vi "Mappa Aplus into WT cluster.vi"(11 "Cluster in":T2) -> (3 "MISURE WT":T1)   [LabVIEW 2019]
uses:
  TypeDef/MISURE WT.ctl
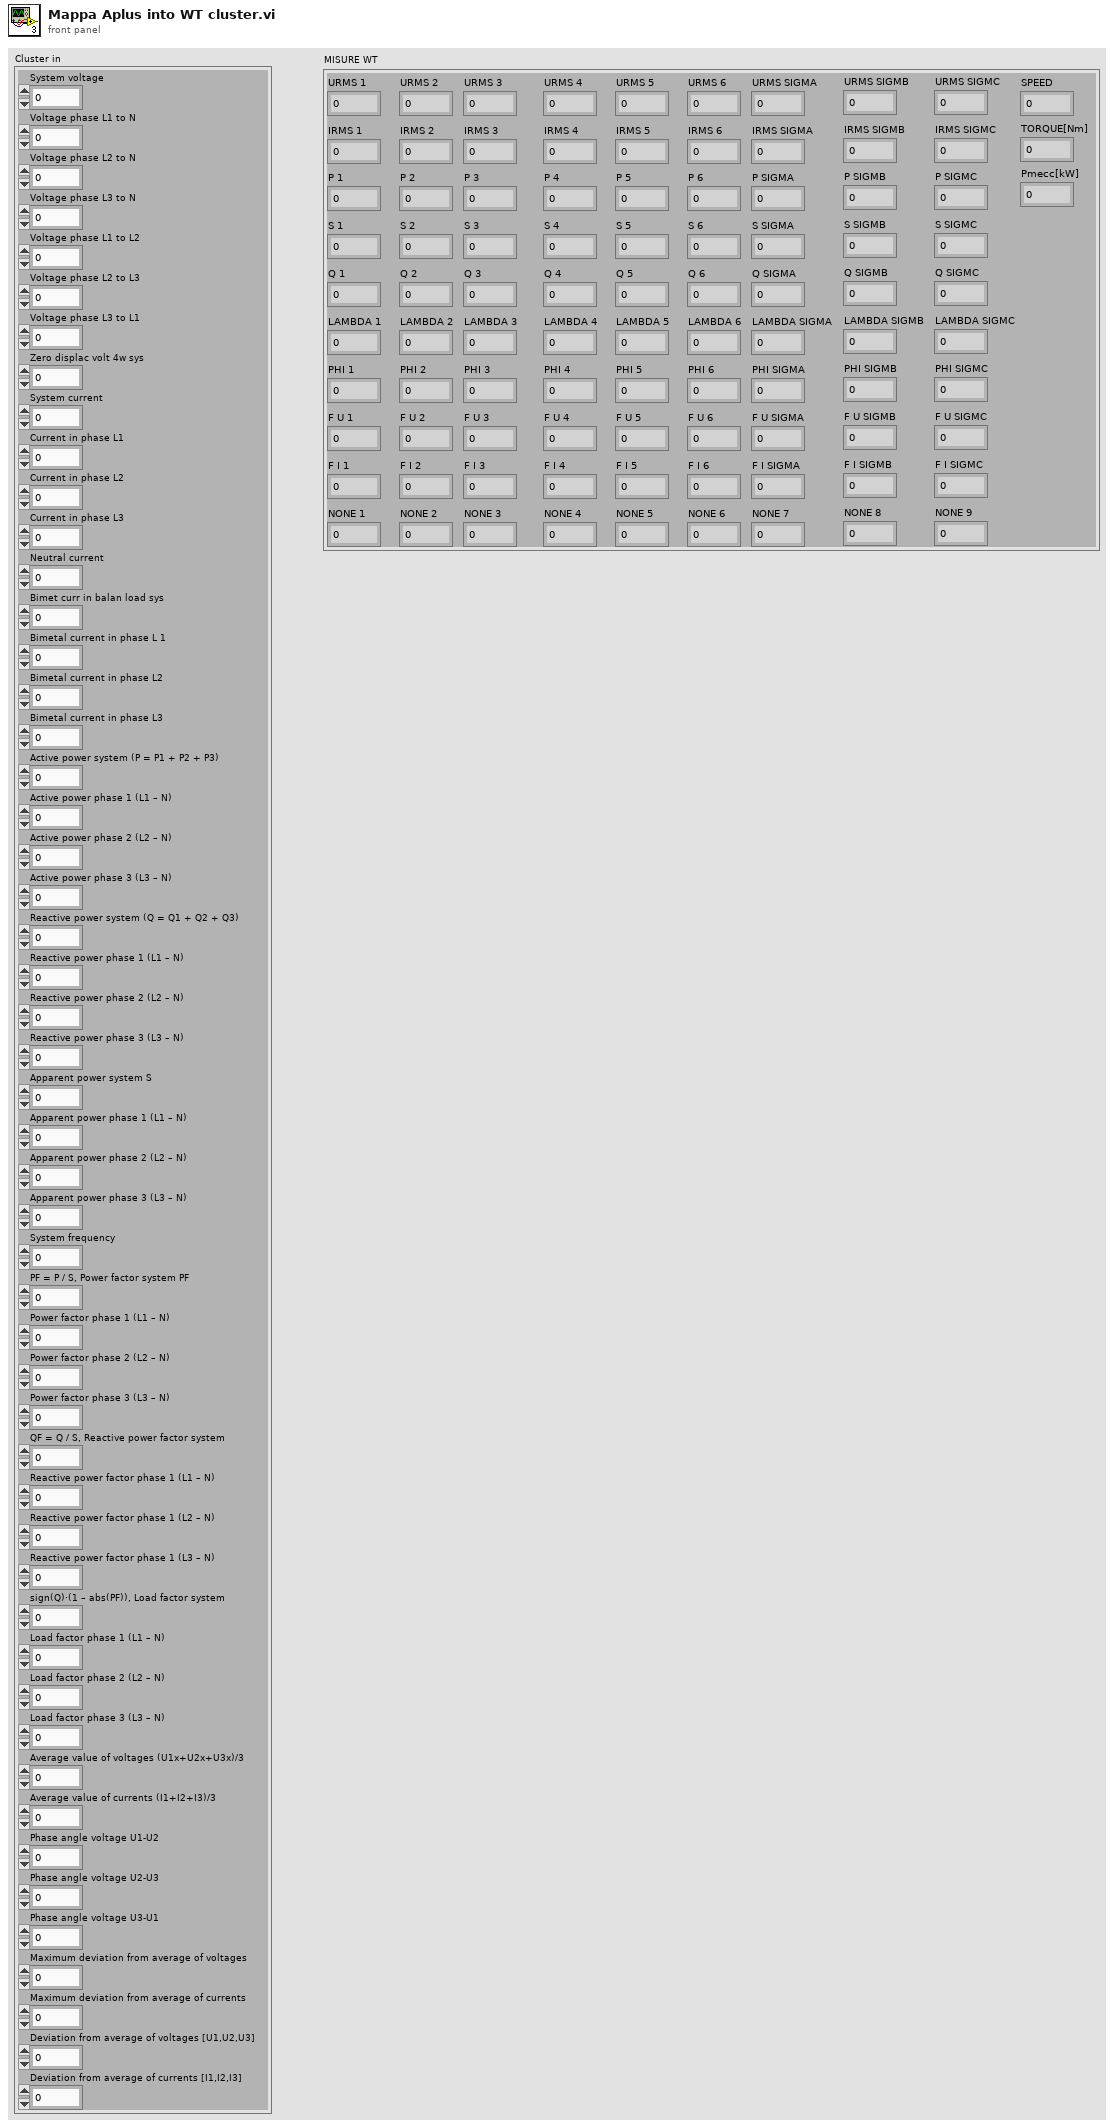
[diagram p1: front panel]
types:
  T1 = typedef "MISURE WT.ctl" = cluster{"URMS 1":dbl, "IRMS 1":dbl, "P 1":dbl, "S 1":dbl, "Q 1":dbl, "LAMBDA 1":dbl, "PHI 1":dbl, "F U 1":dbl, "F I 1":dbl, "NONE 1":dbl, "URMS 2":dbl, "IRMS 2":dbl, "P 2":dbl, "S 2":dbl, "Q 2":dbl, "LAMBDA 2":dbl, "PHI 2":dbl, "F U 2":dbl, "F I 2":dbl, "NONE 2":dbl, "URMS 3":dbl, "IRMS 3":dbl, "P 3":dbl, "S 3":dbl, "Q 3":dbl, "LAMBDA 3":dbl, "PHI 3":dbl, "F U 3":dbl, "F I 3":dbl, "NONE 3":dbl, "URMS 4":dbl, "IRMS 4":dbl, "P 4":dbl, "S 4":dbl, "Q 4":dbl, "LAMBDA 4":dbl, "PHI 4":dbl, "F U 4":dbl, "F I 4":dbl, "NONE 4":dbl, "URMS 5":dbl, "IRMS 5":dbl, "P 5":dbl, "S 5":dbl, "Q 5":dbl, "LAMBDA 5":dbl, "PHI 5":dbl, "F U 5":dbl, "F I 5":dbl, "NONE 5":dbl, "URMS 6":dbl, "IRMS 6":dbl, "P 6":dbl, "S 6":dbl, "Q 6":dbl, "LAMBDA 6":dbl, "PHI 6":dbl, "F U 6":dbl, "F I 6":dbl, "NONE 6":dbl, "URMS SIGMA":dbl, "IRMS SIGMA":dbl, "P SIGMA":dbl, "S SIGMA":dbl, "Q SIGMA":dbl, "LAMBDA SIGMA":dbl, "PHI SIGMA":dbl, "F U SIGMA":dbl, "F I SIGMA":dbl, "NONE 7":dbl, "URMS SIGMB":dbl, "IRMS SIGMB":dbl, "P SIGMB":dbl, "S SIGMB":dbl, "Q SIGMB":dbl, "LAMBDA SIGMB":dbl, "PHI SIGMB":dbl, "F U SIGMB":dbl, "F I SIGMB":dbl, "NONE 8":dbl, "URMS SIGMC":dbl, "IRMS SIGMC":dbl, "P SIGMC":dbl, "S SIGMC":dbl, "Q SIGMC":dbl, "LAMBDA SIGMC":dbl, "PHI SIGMC":dbl, "F U SIGMC":dbl, "F I SIGMC":dbl, "NONE 9":dbl, "SPEED":dbl, "TORQUE[Nm]":dbl, "Pmecc[kW]":dbl}
  T2 = cluster{"System voltage":dbl, "Voltage phase L1 to N":dbl, "Voltage phase L2 to N":dbl, "Voltage phase L3 to N":dbl, "Voltage phase L1 to L2":dbl, "Voltage phase L2 to L3":dbl, "Voltage phase L3 to L1":dbl, "Zero displac volt 4w sys":dbl, "System current":dbl, "Current in phase L1":dbl, "Current in phase L2":dbl, "Current in phase L3":dbl, "Neutral current":dbl, "Bimet curr in balan load sys":dbl, "Bimetal current in phase L 1":dbl, "Bimetal current in phase L2":dbl, "Bimetal current in phase L3":dbl, "Active power system (P = P1 + P2 + P3)":dbl, "Active power phase 1 (L1 – N)":dbl, "Active power phase 2 (L2 – N)":dbl, "Active power phase 3 (L3 – N)":dbl, "Reactive power system (Q = Q1 + Q2 + Q3)":dbl, "Reactive power phase 1 (L1 – N)":dbl, "Reactive power phase 2 (L2 – N)":dbl, "Reactive power phase 3 (L3 – N)":dbl, "Apparent power system S":dbl, "Apparent power phase 1 (L1 – N)":dbl, "Apparent power phase 2 (L2 – N)":dbl, "Apparent power phase 3 (L3 – N)":dbl, "System frequency":dbl, "PF = P / S, Power factor system PF":dbl, "Power factor phase 1 (L1 – N)":dbl, "Power factor phase 2 (L2 – N)":dbl, "Power factor phase 3 (L3 – N)":dbl, "QF = Q / S, Reactive power factor system":dbl, "Reactive power factor phase 1 (L1 – N)":dbl, "Reactive power factor phase 1 (L2 – N)":dbl, "Reactive power factor phase 1 (L3 – N)":dbl, "sign(Q)·(1 – abs(PF)), Load factor system":dbl, "Load factor phase 1 (L1 – N)":dbl, "Load factor phase 2 (L2 – N)":dbl, "Load factor phase 3 (L3 – N)":dbl, "Average value of voltages (U1x+U2x+U3x)/3":dbl, "Average value of currents (I1+I2+I3)/3":dbl, "Phase angle voltage U1-U2":dbl, "Phase angle voltage U2-U3":dbl, "Phase angle voltage U3-U1":dbl, "Maximum deviation from average of voltages":dbl, "Maximum deviation from average of currents":dbl, "Deviation from average of voltages [U1,U2,U3]":dbl, "Deviation from average of currents [I1,I2,I3]":dbl}
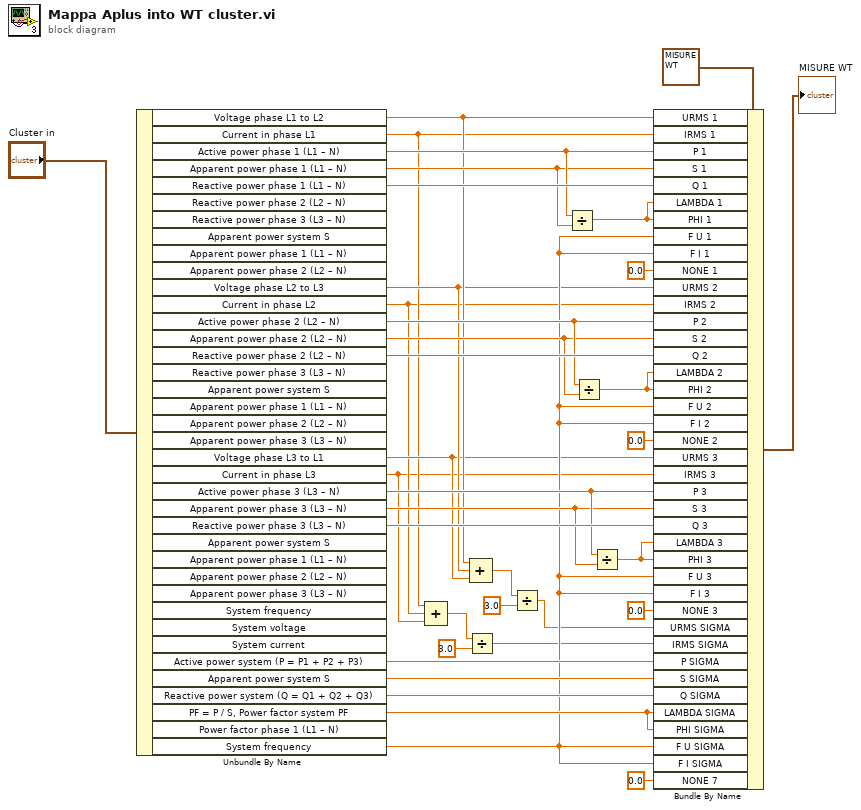
[diagram p0: block diagram]
diagram:
  n1 = Unbundle By Name("Cluster in") -> ("Voltage phase L1 to L2"=w12:dbl, "Current in phase L1"=w3:dbl, "Active power phase 1 (L1 – N)"=w32:dbl, "Apparent power phase 1 (L1 – N)"=w31:dbl, "Reactive power phase 1 (L1 – N)"=w33:dbl, "Voltage phase L2 to L3"=w11:dbl, "Current in phase L2"=w2:dbl, "Active power phase 2 (L2 – N)"=w29:dbl, "Apparent power phase 2 (L2 – N)"=w28:dbl, "Reactive power phase 2 (L2 – N)"=w30:dbl, "Voltage phase L3 to L1"=w10:dbl, "Current in phase L3"=w1:dbl, "Active power phase 3 (L3 – N)"=w26:dbl, "Apparent power phase 3 (L3 – N)"=w25:dbl, "Reactive power phase 3 (L3 – N)"=w27:dbl, "Active power system (P = P1 + P2 + P3)"=w24:dbl, "Apparent power system S"=w23:dbl, "Reactive power system (Q = Q1 + Q2 + Q3)"=w22:dbl, "PF = P / S, Power factor system PF"=w21:dbl, "System frequency"=w17:dbl)  [unwired: 18 out]
  n2 = Compound Arithmetic op=ADD(w3, w2, w1) -> (w5:dbl)
  n3 = Divide(x=w5, y=3.0) -> (x/y=w4:dbl)
  n4 = Compound Arithmetic op=ADD(w12, w11, w10) -> (w9:dbl)
  n5 = Divide(x=w9, y=3.0) -> (x/y=w7:dbl)
  n6 = Divide(x=w32, y=w31) -> (x/y=w20:dbl)
  n7 = Divide(x=w29, y=w28) -> (x/y=w19:dbl)
  n8 = Divide(x=w26, y=w25) -> (x/y=w18:dbl)
  n9 = Bundle By Name(cluster=T1 {"URMS 1"=0.0, "IRMS 1"=0.0, "P 1"=0.0, "S 1"=0.0, "Q 1"=0.0, "LAMBDA 1"=0.0, "PHI 1"=0.0, "F U 1"=0.0, "F I 1"=0.0, "NONE 1"=0.0, "URMS 2"=0.0, "IRMS 2"=0.0, "P 2"=0.0, "S 2"=0.0, "Q 2"=0.0, "LAMBDA 2"=0.0, "PHI 2"=0.0, "F U 2"=0.0, "F I 2"=0.0, "NONE 2"=0.0, "URMS 3"=0.0, "IRMS 3"=0.0, "P 3"=0.0, "S 3"=0.0, "Q 3"=0.0, "LAMBDA 3"=0.0, "PHI 3"=0.0, "F U 3"=0.0, "F I 3"=0.0, "NONE 3"=0.0, "URMS 4"=0.0, "IRMS 4"=0.0, "P 4"=0.0, "S 4"=0.0, "Q 4"=0.0, "LAMBDA 4"=0.0, "PHI 4"=0.0, "F U 4"=0.0, "F I 4"=0.0, "NONE 4"=0.0, "URMS 5"=0.0, "IRMS 5"=0.0, "P 5"=0.0, "S 5"=0.0, "Q 5"=0.0, "LAMBDA 5"=0.0, "PHI 5"=0.0, "F U 5"=0.0, "F I 5"=0.0, "NONE 5"=0.0, "URMS 6"=0.0, "IRMS 6"=0.0, "P 6"=0.0, "S 6"=0.0, "Q 6"=0.0, "LAMBDA 6"=0.0, "PHI 6"=0.0, "F U 6"=0.0, "F I 6"=0.0, "NONE 6"=0.0, "URMS SIGMA"=0.0, "IRMS SIGMA"=0.0, "P SIGMA"=0.0, "S SIGMA"=0.0, "Q SIGMA"=0.0, "LAMBDA SIGMA"=0.0, "PHI SIGMA"=0.0, "F U SIGMA"=0.0, "F I SIGMA"=0.0, "NONE 7"=0.0, "URMS SIGMB"=0.0, "IRMS SIGMB"=0.0, "P SIGMB"=0.0, "S SIGMB"=0.0, "Q SIGMB"=0.0, "LAMBDA SIGMB"=0.0, "PHI SIGMB"=0.0, "F U SIGMB"=0.0, "F I SIGMB"=0.0, "NONE 8"=0.0, "URMS SIGMC"=0.0, "IRMS SIGMC"=0.0, "P SIGMC"=0.0, "S SIGMC"=0.0, "Q SIGMC"=0.0, "LAMBDA SIGMC"=0.0, "PHI SIGMC"=0.0, "F U SIGMC"=0.0, "F I SIGMC"=0.0, "NONE 9"=0.0, "SPEED"=0.0, "TORQUE[Nm]"=0.0, "Pmecc[kW]"=0.0} ("MISURE WT"), "URMS 1"=w12, "IRMS 1"=w3, "P 1"=w32, "S 1"=w31, "Q 1"=w33, "LAMBDA 1"=w20, "PHI 1"=w20, "F U 1"=w17, "F I 1"=w17, "NONE 1"=0.0, "URMS 2"=w11, "IRMS 2"=w2, "P 2"=w29, "S 2"=w28, "Q 2"=w30, "LAMBDA 2"=w19, "PHI 2"=w19, "F U 2"=w17, "F I 2"=w17, "NONE 2"=0.0, "URMS 3"=w10, "IRMS 3"=w1, "P 3"=w26, "S 3"=w25, "Q 3"=w27, "LAMBDA 3"=w18, "PHI 3"=w18, "F U 3"=w17, "F I 3"=w17, "NONE 3"=0.0, "URMS SIGMA"=w7, "IRMS SIGMA"=w4, "P SIGMA"=w24, "S SIGMA"=w23, "Q SIGMA"=w22, "LAMBDA SIGMA"=w21, "PHI SIGMA"=w21, "F U SIGMA"=w17, "F I SIGMA"=w17, "NONE 7"=0.0) -> (→"MISURE WT":T1)
